vi "ENAclose.vi"(1 "Error In (no error)":errorcluster, 2 "VISA session":refnum<visa-resource-name>) -> (0 "Error Out":errorcluster)   [LabVIEW 2017]
uses:
  <instrlib>/Agilent ENA Series/Agilent ENA Series.lvlib
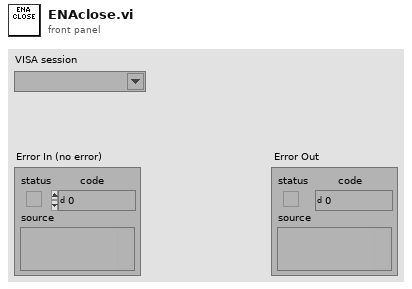
[diagram p1: front panel]
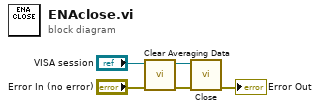
[diagram p0: block diagram]
diagram:
  n1 = call <instrlib>:"Clear Averaging Data.vi"("error in (no error)"="Error In (no error)", "VISA resource name"="VISA session") -> ("error out"=w4:errorcluster, "VISA resource name out"=w5:refnum<visa-resource-name>)  [unwired: 8 in]
  n2 = call <instrlib>:"Close.vi"("error in (no error)"=w4, "VISA resource name"=w5) -> ("error out"=→"Error Out":errorcluster)  [unwired: 9 in]
